vi "PWM Value to Voltage Conversion.vi"(10 "PWM":dbl) -> (2 "Voltage":dbl)   [LabVIEW 2011]
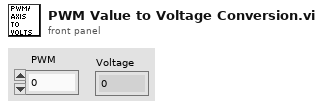
[diagram p1: front panel]
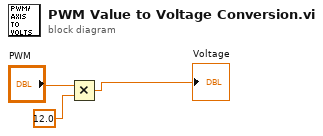
[diagram p0: block diagram]
diagram:
  n1 = Multiply(x="PWM", y=12.0) -> (x*y=→"Voltage":dbl)
